vi "RUS Sweep -- get thermometer snapshot.vi"(8 "error in (no error)":errorcluster, 11 "thermometers in":T1={"ITC Temperature"=0.0, "ITC Set Temperature"=0.0, "LTC Temperature"=0.0, "LTC21 Address"="GPIB0::15::INSTR", "ITC503 Address"="GPIB0::24::INSTR"}) -> (0 "error out":errorcluster={"status"=TRUE, "code"=-200019, "source"="DAQmx Read (Analog 1D Wfm NChan NSamp).vi:1<append>\n<B>Task Name: </B>_unnamedTask<2C36>"}, 3 "thermometers out":T1={"ITC Temperature"=0.0, "ITC Set Temperature"=0.0, "LTC Temperature"=0.0, "LTC21 Address"="GPIB0::15::INSTR", "ITC503 Address"="GPIB0::24::INSTR"})   [LabVIEW 2010]
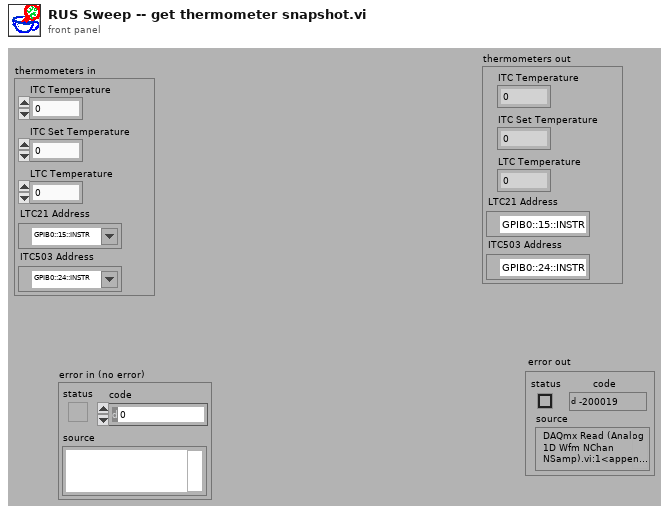
[diagram p1: front panel]
types:
  T1 = cluster{"ITC Temperature":dbl, "ITC Set Temperature":dbl, "LTC Temperature":dbl, "LTC21 Address":refnum<visa-resource-name>, "ITC503 Address":refnum<visa-resource-name>}
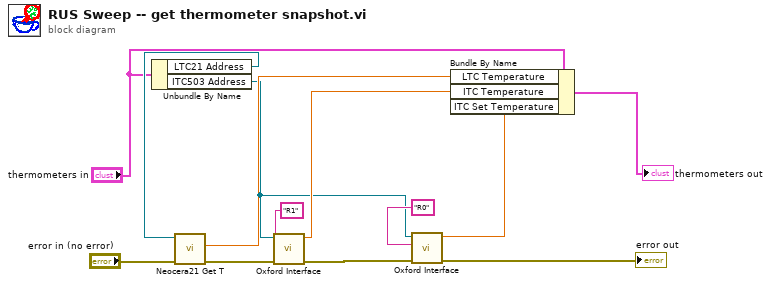
[diagram p0: block diagram]
diagram:
  n1 = Unbundle By Name("thermometers in") -> ("LTC21 Address"=w8:refnum<visa-resource-name>, "ITC503 Address"=w1:refnum<visa-resource-name>)
  n2 = call "Neocera21 Get T.vi"("error in (no error)"="error in (no error)", "VISA Resource Name"=w8) -> ("error out"=w13:errorcluster, "Temperature"=w6:dbl)  [unwired: 6 in, 2 out]
  n3 = call "Oxford Interface.vi"("error in (no error)"=w13, "Command"="R1", "Address"=w1) -> ("error out"=w11:errorcluster, "Numeric reply"=w4:dbl)  [unwired: 7 out]
  n4 = call "Oxford Interface.vi"("error in (no error)"=w11, "Command"="R0", "Address"=w1) -> ("error out"=→"error out":errorcluster, "Numeric reply"=w3:dbl)  [unwired: 7 out]
  n5 = Bundle By Name(cluster="thermometers in", "LTC Temperature"=w6, "ITC Temperature"=w4, "ITC Set Temperature"=w3) -> (→"thermometers out":T1)
